vi "Close Vi Reference.vi"(8 "error in (no error)":errorcluster, 11 "reference":refnum<vi>) -> (0 "error out":errorcluster, 3 "reference out":refnum<vi>)   [LabVIEW 2011]
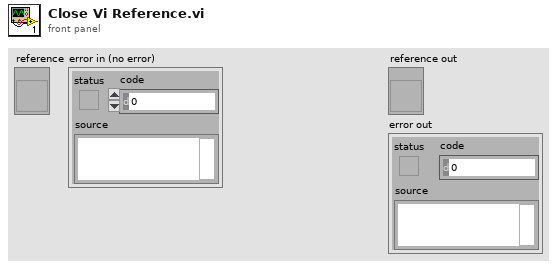
[diagram p1: front panel]
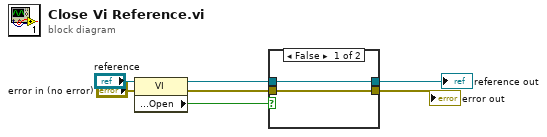
[diagram p0: block diagram]
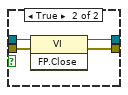
[diagram p2: hidden frame]
diagram:
  n1 = property class="VI"(reference="reference", error in="error in (no error)") -> (reference out=w7:refnum<vi>, error out=w6:errorcluster, "Front Panel.Open"=w5:bool)
  n2 = case shown="False" w5 {
    tunnel: w7 -> [w9 w13]
    tunnel: w6 -> [w8 w12]
    tunnel: [w9 w11] -> w2
    tunnel: [w8 w10] -> w1
    frame False {
    }
    frame True {
      n3 = invoke class="VI" method="FP.Close"(reference=w13, error in=w12) -> (reference out=w11:refnum<vi>, error out=w10:errorcluster)  [unwired: 1 in, 1 out]
    }
  }
  "reference out" <- w2
  "error out" <- w1
